vi "IconlibraryStuffInProgress.vi"(6 "Abort Button Text (\"\")":string, 7 "FP.Title":string, 8 "error in (no error)":errorcluster, 9 "Show FP Timeout (ms)":i32, 10 "Message in":string, 11 "Close Notifier":refnum<notifier>) -> (0 "error out":errorcluster, 1 "Aborted":bool, 3 "Close Notifier out":refnum<notifier>)   [LabVIEW 2020]
panel:
  in  "Abort Button":bool
  out "Progress":u8(slide) scale=0.0..100.0
  out "Message":string
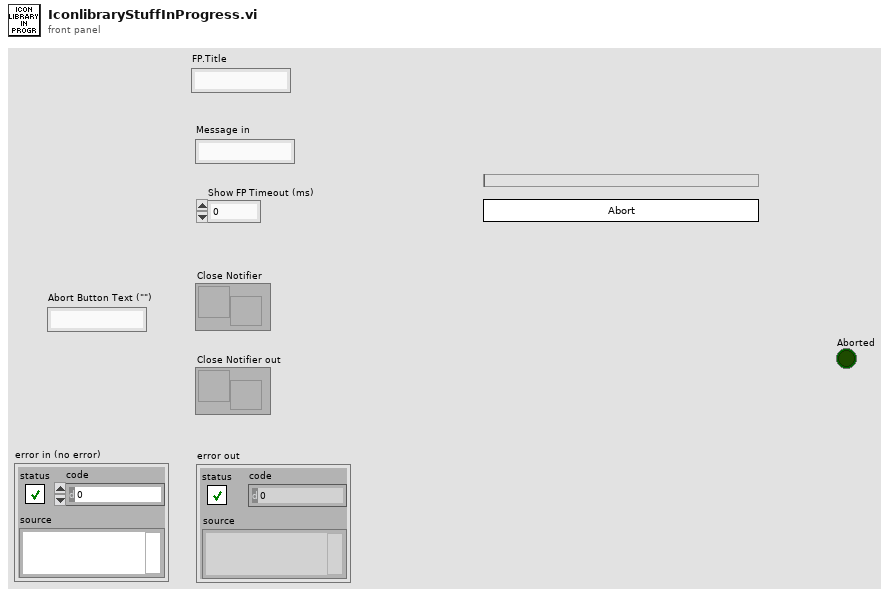
[diagram p1: front panel]
types:
  T1 = typedef "LVRectTypeDef.ctl" = cluster{"Left":i16, "Top":i16, "Right":i16, "Bottom":i16}
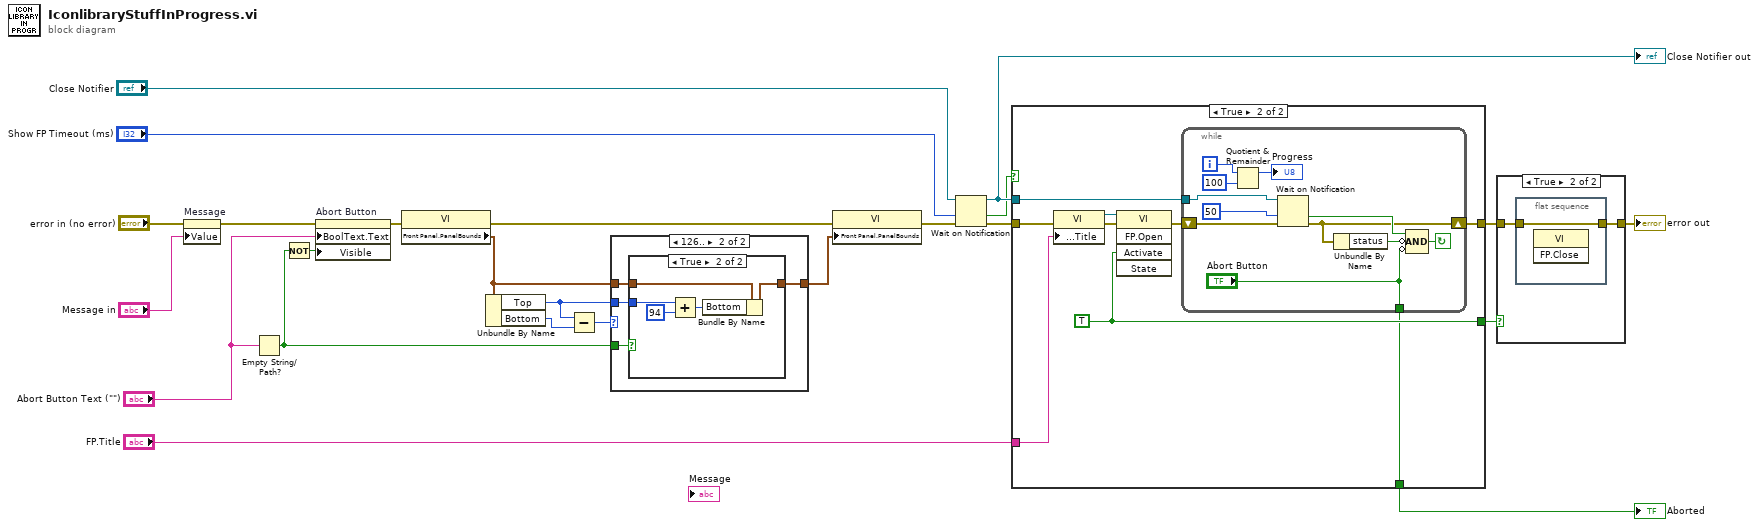
[diagram p0: block diagram]
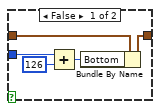
[diagram p3: hidden frame]
diagram:
  n1 = property on="Message" class="Str"(error in="error in (no error)", "Value"="Message in") -> (error out=w13:errorcluster)  [unwired: 1 in, 1 out]
  n2 = Empty String/Path?(string/path="Abort Button Text (\"\")") -> (empty?=w4:bool)
  n3 = Not(x=w4) -> (.not. x?=w12:bool)
  n4 = property on="Abort Button" class="Bool"(error in=w13, "BoolText.Text"="Abort Button Text (\"\")", "Visible"=w12) -> (error out=w10:errorcluster)  [unwired: 1 in, 1 out]
  n5 = property class="VI"(error in=w10) -> (error out=w7:errorcluster, "Front Panel.PanelBounds"=w5:T1)  [unwired: 1 in, 1 out]
  n6 = Unbundle By Name(w5) -> ("Top"=w2:i16, "Bottom"=w9:i16)
  n7 = Subtract(x=w2, y=w9) -> (x-y=w8:i16)
  n8 = case shown="126.." w8 {
    tunnel: w5 -> [w26 w37]
    tunnel: w4 -> [w28 w38]
    tunnel: [w27 w35] -> w3
    tunnel: w2 -> [w25 w36]
    frame 0, Default {
      n9 = case shown="True" w28 {
        tunnel: [w30 w34] -> w27
        tunnel: w26 -> [w31 w34]
        tunnel: w25 -> [w33 _]
        frame False {
          n10 = Add(x=w33, y=i16 126) -> (x+y=w29:i16)
          n11 = Bundle By Name(cluster=w31, "Bottom"=w29) -> (w30:T1)
        }
        frame True {
        }
      }
    }
    frame 126.. {
      n12 = case shown="True" w38 {
        tunnel: w37 -> [w39 w44]
        tunnel: w36 -> [_ w43]
        tunnel: [w39 w40] -> w35
        frame False {
        }
        frame True {
          n13 = Add(x=w43, y=i16 94) -> (x+y=w41:i16)
          n14 = Bundle By Name(cluster=w44, "Bottom"=w41) -> (w40:T1)
        }
      }
    }
  }
  n15 = property class="VI"(error in=w7, "Front Panel.PanelBounds"=w3) -> (error out=w6:errorcluster)  [unwired: 1 in, 1 out]
  n16 = Wait on Notification(notifier="Close Notifier", timeout in ms (-1)="Show FP Timeout (ms)", error in (no error)=w6) -> (notifier out=w17:refnum<notifier>, timed out?=w14:bool, error out=w16:errorcluster)  [unwired: 2 out]
  "Close Notifier out" <- w17
  n17 = case shown="True" w14 {
    tunnel: w17 -> [_ w54]
    tunnel: [_ w53] -> w23
    tunnel: [w45 w47] -> w21
    tunnel: "FP.Title" -> [_ w50]
    tunnel: w16 -> [w45 w49]
    tunnel: [_ w46] -> w1
    frame False {
    }
    frame True {
      w53 = TRUE ("Activate?")
      n18 = property class="VI"(error in=w49, "Front Panel.Title"=w50) -> (reference out=w52:refnum<vi>, error out=w51:errorcluster)  [unwired: 1 in]
      n19 = invoke class="VI" method="FP.Open"(reference=w52, error in=w51, "Activate"=w53) -> (error out=w48:errorcluster)  [unwired: 2 in, 4 out]
      n20 = while {
        tunnel: w54 -> [w62]
        shift-right: [w56] -> w47
        shift-left: w48 -> [w59]
        tunnel: ["Abort Button"] -> w46
        i -> [w65]
        stop <- w58 continue-if-true
        n21 = Quotient & Remainder(x=w65, y=100) -> (x-y*floor(x/y)=→"Progress":i32)  [unwired: 1 out]
        n22 = Wait on Notification(notifier=w62, timeout in ms (-1)=50 ("ms timeout (-1)"), error in (no error)=w59) -> (timed out?=w60:bool, error out=w56:errorcluster)  [unwired: 3 out]
        n23 = Unbundle By Name(w56) -> ("status"=w57:bool)
        n24 = Compound Arithmetic op=AND(w60, invert w57, invert "Abort Button") -> (w58:bool)
      }
    }
  }
  "Aborted" <- w1
  n25 = case shown="True" w23 {
    tunnel: w21 -> [w66 w67]
    tunnel: [w66 w68] -> w15
    frame False {
    }
    frame True {
      n26 = flat-sequence {
        tunnel: [w69] -> w68
        tunnel: w67 -> [w69]
        frame #0 {
          n27 = invoke class="VI" method="FP.Close"() -> ()  [unwired: 3 in, 3 out]
        }
      }
    }
  }
  "error out" <- w15
